vi "2024_day10_RescoursiveSearch(SubVI).vi"(8 "Trailheads In":string[](array[string]), 9 "Topographic Map":i32[][](array[numeric]), 10 "Start Column":i32, 11 "Start Row":i32) -> (0 "Trailheads Out":string[](array[string]))   [LabVIEW 2023]
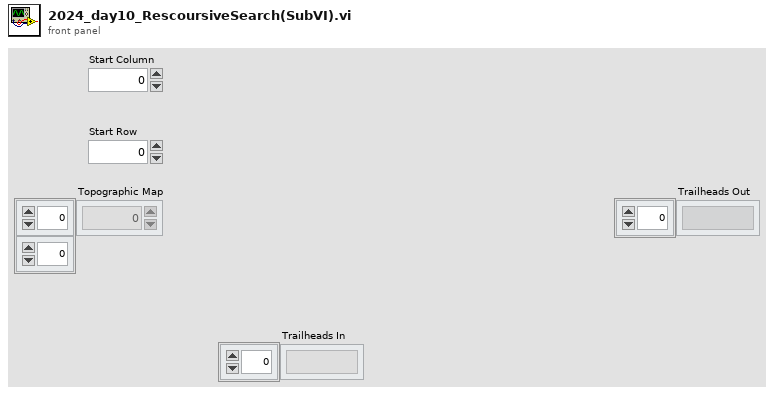
[diagram p1: front panel]
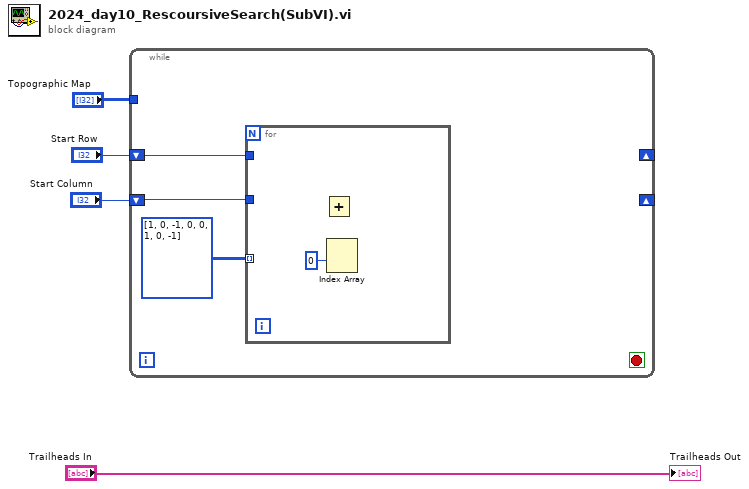
[diagram p0: block diagram]
diagram:
  n1 = while {
    tunnel: "Topographic Map" -> [_]
    shift-right: _ -> [_]
    shift-left: "Start Row" -> [w7]
    shift-right: _ -> [_]
    shift-left: "Start Column" -> [w6]
    stop <- _ stop-if-true
    n2 = for {
      tunnel: w7 -> [_]
      tunnel: w6 -> [_]
      tunnel: i32[][] [[1, 0], [-1, 0], [0, 1], [0, -1]] -> [_] mode=indexing
      n3 = Add() -> ()  [unwired: 2 in, 1 out]
      n4 = Index Array(index #1=0 ("index")) -> ()  [unwired: 2 in, 2 out]
    }
  }
  "Trailheads Out" <- "Trailheads In"
